vi "UnitTest-CheckForEveryIntervalGiven.vi"(8 "error in (no error)":errorcluster) -> (0 "error out":errorcluster)   [LabVIEW 2014]
uses:
  TableLogger_Actor/TableLoggerConfig.ctl
  TableLogger_Actor/TableLoggerTypes.ctl
  TableLogger_Actor/TableLoggerBackupConfig.ctl
  <vilib>/addons/_JKI Toolkits/Caraya/classes/Test/Test.lvclass
  <vilib>/addons/_JKI Toolkits/Caraya/classes/Assert/Assert.lvclass
  TableLogger_Actor/TableLogger_Actor.lvlib
panel:
  # "Connector Pane"
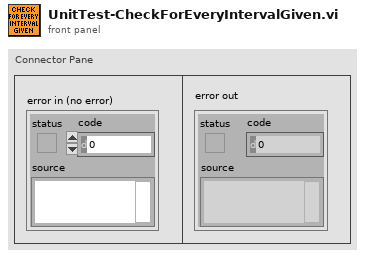
[diagram p1: front panel]
types:
  T1 = typedef "TableLogger_Actor.lvlib/TableLoggerConfig.ctl" = cluster{"TableLogger":T2, "DB File Path":path, "DB Backup Config":T3}
  T2 = typedef "TableLogger_Actor.lvlib/TableLoggerTypes.ctl" = enum16{"CSV Logger", "SQLite Logger"}
  T3 = typedef "TableLogger_Actor.lvlib/TableLoggerBackupConfig.ctl" = cluster{"Directory":path, "UTC Time Format":bool, "On Launch":bool, "Interval (Hours)":dbl, "Size Multiples (Bytes)":i32}
  T4 = typedef "TableLogger_Actor.lvlib/TableLoggerDataCluster.ctl" = cluster{"Numeric Data":i32, "Float Data":dbl, "String Data":string, "Enum Data":enum16{"Enum Item 1", "Enum Item 2"}, "Array Data":i32[]}
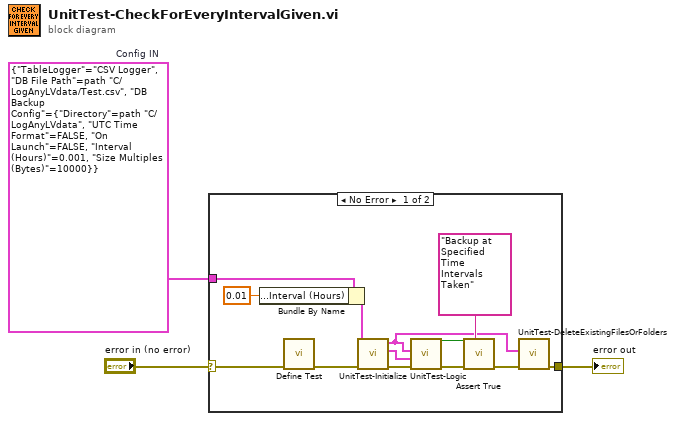
[diagram p0: block diagram]
diagram:
  w1 = T1 {"TableLogger"=enum."CSV Logger", "DB File Path"=path "C:/LogAnyLVdata/Test.csv", "DB Backup Config"={"Directory"=path "C:/LogAnyLVdata", "UTC Time Format"=FALSE, "On Launch"=FALSE, "Interval (Hours)"=0.001, "Size Multiples (Bytes)"=10000}}  # Config IN
  n1 = case shown="No Error" "error in (no error)" {
    selector: "error in (no error)" -> [w16 w17]
    tunnel: [w11 w17] -> w2
    tunnel: w1 -> [w8 _]
    frame No Error {
      n2 = Bundle By Name(cluster=w8, "DB Backup Config.Interval (Hours)"=0.01) -> (w5:T1)
      n3 = call <vilib>:"Define Test.vi"("error in (no error)"=w16) -> ("error out"=w14:errorcluster)  [unwired: 10 in]
      n4 = call "UnitTest-Initialize.vi"("error in"=w14, "Config IN"=w5) -> ("error out"=w13:errorcluster, "LV Data"=w12:T4, "Config OUT"=w6:T1)  [unwired: 7 in]
      n5 = call "UnitTest-Logic.vi"("error in (no error)"=w13, "LV Data"=w12, "TableLogger Config"=w6) -> ("error out"=w10:errorcluster, "Test Result"=w7:bool)  [unwired: 7 in]
      n6 = call <vilib>:"Assert True.vi"("Label"="Backup at Specified Time Intervals Taken", "error in (no error)"=w10, "True?"=w7) -> ("error out"=w9:errorcluster)  [unwired: 8 in]
      n7 = call "UnitTest-DeleteExistingFilesOrFolders.vi"("error in (no error)"=w9, "Config IN"=w6) -> ("error out"=w11:errorcluster)  [unwired: 9 in]
    }
    frame Error {
    }
  }
  "error out" <- w2
